vi "Configure9206.vi"(7 "Channel Number":i32, 8 "error in (no error)":errorcluster, 10 "Properties":T1[](array[typedef]), 11 "IO Ref in":refnum<k21>) -> (0 "error out":errorcluster, 3 "IO Ref out":refnum<k21>)   [LabVIEW 2017, in "ScanEngine.lvlib"]
uses:
  <vilib>/addons/InsightCM/Devices/Shared/Common/ScanEngine/ScanEngine.lvlib
  <vilib>/addons/InsightCM/MessageBus/Base/controls/KeyValuePair.ctl
  <resource>/objmgr/cRIO.rc
  <vilib>/addons/InsightCM/Utilities/PropertyHelpers/PropertyHelpers.lvlib
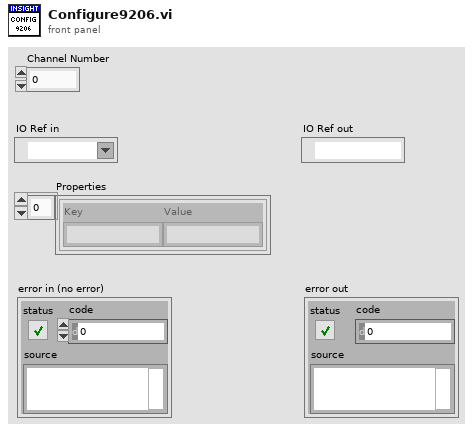
[diagram p1: front panel]
types:
  T1 = typedef "KeyValuePair.ctl" = cluster{"Key":string, "Value":string}
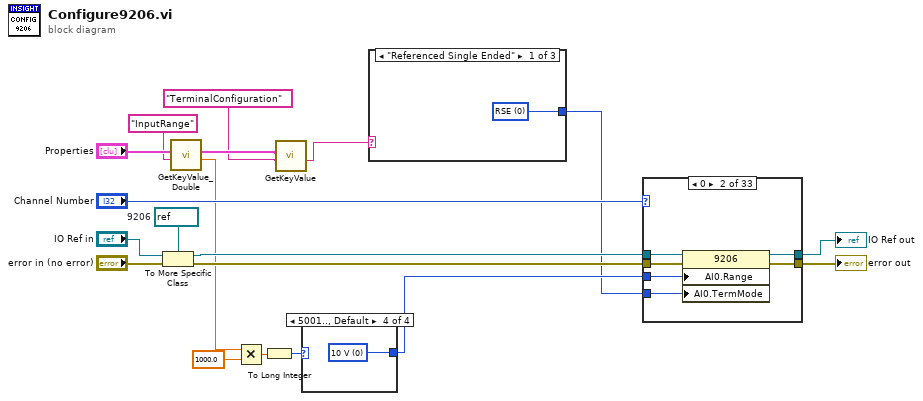
[diagram p0: block diagram]
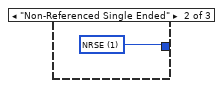
[diagram p2: hidden frame]
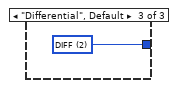
[diagram p3: hidden frame]
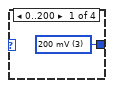
[diagram p4: hidden frame]
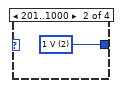
[diagram p5: hidden frame]
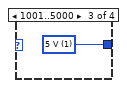
[diagram p6: hidden frame]
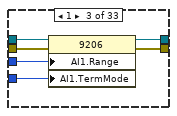
[diagram p8: hidden frame]
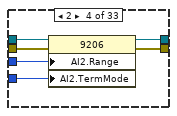
[diagram p9: hidden frame]
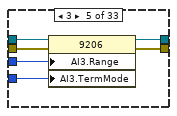
[diagram p10: hidden frame]
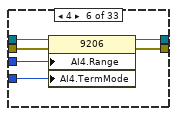
[diagram p11: hidden frame]
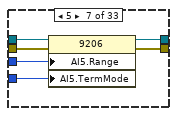
[diagram p12: hidden frame]
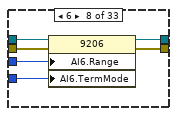
[diagram p13: hidden frame]
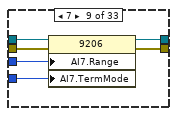
[diagram p14: hidden frame]
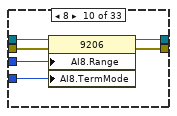
[diagram p15: hidden frame]
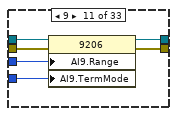
[diagram p16: hidden frame]
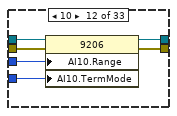
[diagram p17: hidden frame]
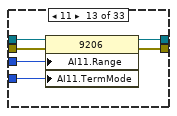
[diagram p18: hidden frame]
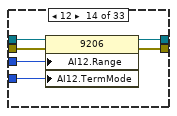
[diagram p19: hidden frame]
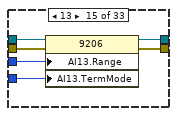
[diagram p20: hidden frame]
diagram:
  w12 = refnum<k21> refnum  # 9206
  n1 = To More Specific Class(target class=w12, reference="IO Ref in", error in="error in (no error)") -> (specific class reference=w11:refnum<k21>, error out=w15:errorcluster)
  n2 = call <vilib>:"GetKeyValue_Double.vi"("key"="InputRange" ("name"), "key value pairs"="Properties") -> ("value"=w5:dbl, "key value pairs out"=w4:T1[])  [unwired: 7 in, 1 out]
  n3 = Multiply(x=w5, y=1000.0) -> (x*y=w17:dbl)
  n4 = To Long Integer(number=w17) -> (32bit integer=w16:i32)
  n5 = call <vilib>:"GetKeyValue.vi"("key"="TerminalConfiguration" ("name"), "key value pairs"=w4) -> ("value"=w2:string)  [unwired: 7 in, 2 out]
  n6 = case shown="5001.., Default" w16 {
    tunnel: [w20 w21 w22 w23] -> w19
    frame 0..200 {
      w20 = u32 3 items=["10 V", "5 V", "1 V", "200 mV"] ("9205 Range")
    }
    frame 201..1000 {
      w21 = u32 2 items=["10 V", "5 V", "1 V", "200 mV"] ("9205 Range")
    }
    frame 1001..5000 {
      w22 = u32 1 items=["10 V", "5 V", "1 V", "200 mV"] ("9205 Range")
    }
    frame 5001.., Default {
      w23 = u32 0 items=["10 V", "5 V", "1 V", "200 mV"] ("9205 Range")
    }
  }
  n7 = case shown="\"Referenced Single Ended\"" w2 {
    tunnel: [w24 w25 w26] -> w1
    frame "Referenced Single Ended" {
      w24 = u32 0 items=["RSE", "NRSE", "DIFF"] ("AI0:Terminal mode")
    }
    frame "Non-Referenced Single Ended" {
      w25 = u32 1 items=["RSE", "NRSE", "DIFF"] ("AI0:Terminal mode")
    }
    frame "Differential", Default {
      w26 = u32 2 items=["RSE", "NRSE", "DIFF"] ("AI0:Terminal mode")
    }
  }
  n8 = case shown="0" "Channel Number" {
    tunnel: w15 -> [w28 w34 w40 w46 w52 w58 w64 w70 w76 w82 w88 w94 w100 w106 w112 w118 w124 w130 w136 w142 w148 w154 w160 w166 w172 w178 w184 w190 w196 w202 w208 w214 w220]
    tunnel: [w28 w33 w39 w45 w51 w57 w63 w69 w75 w81 w87 w93 w99 w105 w111 w117 w123 w129 w135 w141 w147 w153 w159 w165 w171 w177 w183 w189 w195 w201 w207 w213 w219] -> w8
    tunnel: w11 -> [w27 w32 w38 w44 w50 w56 w62 w68 w74 w80 w86 w92 w98 w104 w110 w116 w122 w128 w134 w140 w146 w152 w158 w164 w170 w176 w182 w188 w194 w200 w206 w212 w218]
    tunnel: [w27 w31 w37 w43 w49 w55 w61 w67 w73 w79 w85 w91 w97 w103 w109 w115 w121 w127 w133 w139 w145 w151 w157 w163 w169 w175 w181 w187 w193 w199 w205 w211 w217] -> w13
    tunnel: w1 -> [_ w30 w36 w42 w48 w54 w60 w66 w72 w78 w84 w90 w96 w102 w108 w114 w120 w126 w132 w138 w144 w150 w156 w162 w168 w174 w180 w186 w192 w198 w204 w210 w216]
    tunnel: w19 -> [_ w29 w35 w41 w47 w53 w59 w65 w71 w77 w83 w89 w95 w101 w107 w113 w119 w125 w131 w137 w143 w149 w155 w161 w167 w173 w179 w185 w191 w197 w203 w209 w215]
    frame -1, Default {
    }
    frame 0 {
      n9 = property class="9206"(reference=w32, error in=w34, "AI0.Range"=w29, "AI0.TermMode"=w30) -> (reference out=w31:refnum<k21>, error out=w33:errorcluster)
    }
    frame 1 {
      n10 = property class="9206"(reference=w38, error in=w40, "AI1.Range"=w35, "AI1.TermMode"=w36) -> (reference out=w37:refnum<k21>, error out=w39:errorcluster)
    }
    frame 2 {
      n11 = property class="9206"(reference=w44, error in=w46, "AI2.Range"=w41, "AI2.TermMode"=w42) -> (reference out=w43:refnum<k21>, error out=w45:errorcluster)
    }
    frame 3 {
      n12 = property class="9206"(reference=w50, error in=w52, "AI3.Range"=w47, "AI3.TermMode"=w48) -> (reference out=w49:refnum<k21>, error out=w51:errorcluster)
    }
    frame 4 {
      n13 = property class="9206"(reference=w56, error in=w58, "AI4.Range"=w53, "AI4.TermMode"=w54) -> (reference out=w55:refnum<k21>, error out=w57:errorcluster)
    }
    frame 5 {
      n14 = property class="9206"(reference=w62, error in=w64, "AI5.Range"=w59, "AI5.TermMode"=w60) -> (reference out=w61:refnum<k21>, error out=w63:errorcluster)
    }
    frame 6 {
      n15 = property class="9206"(reference=w68, error in=w70, "AI6.Range"=w65, "AI6.TermMode"=w66) -> (reference out=w67:refnum<k21>, error out=w69:errorcluster)
    }
    frame 7 {
      n16 = property class="9206"(reference=w74, error in=w76, "AI7.Range"=w71, "AI7.TermMode"=w72) -> (reference out=w73:refnum<k21>, error out=w75:errorcluster)
    }
    frame 8 {
      n17 = property class="9206"(reference=w80, error in=w82, "AI8.Range"=w77, "AI8.TermMode"=w78) -> (reference out=w79:refnum<k21>, error out=w81:errorcluster)
    }
    frame 9 {
      n18 = property class="9206"(reference=w86, error in=w88, "AI9.Range"=w83, "AI9.TermMode"=w84) -> (reference out=w85:refnum<k21>, error out=w87:errorcluster)
    }
    frame 10 {
      n19 = property class="9206"(reference=w92, error in=w94, "AI10.Range"=w89, "AI10.TermMode"=w90) -> (reference out=w91:refnum<k21>, error out=w93:errorcluster)
    }
    frame 11 {
      n20 = property class="9206"(reference=w98, error in=w100, "AI11.Range"=w95, "AI11.TermMode"=w96) -> (reference out=w97:refnum<k21>, error out=w99:errorcluster)
    }
    frame 12 {
      n21 = property class="9206"(reference=w104, error in=w106, "AI12.Range"=w101, "AI12.TermMode"=w102) -> (reference out=w103:refnum<k21>, error out=w105:errorcluster)
    }
    frame 13 {
      n22 = property class="9206"(reference=w110, error in=w112, "AI13.Range"=w107, "AI13.TermMode"=w108) -> (reference out=w109:refnum<k21>, error out=w111:errorcluster)
    }
    frame 14 {
      n23 = property class="9206"(reference=w116, error in=w118, "AI14.Range"=w113, "AI14.TermMode"=w114) -> (reference out=w115:refnum<k21>, error out=w117:errorcluster)
    }
    frame 15 {
      n24 = property class="9206"(reference=w122, error in=w124, "AI15.Range"=w119, "AI15.TermMode"=w120) -> (reference out=w121:refnum<k21>, error out=w123:errorcluster)
    }
    frame 16 {
      n25 = property class="9206"(reference=w128, error in=w130, "AI16.Range"=w125, "AI16.TermMode"=w126) -> (reference out=w127:refnum<k21>, error out=w129:errorcluster)
    }
    frame 17 {
      n26 = property class="9206"(reference=w134, error in=w136, "AI17.Range"=w131, "AI17.TermMode"=w132) -> (reference out=w133:refnum<k21>, error out=w135:errorcluster)
    }
    frame 18 {
      n27 = property class="9206"(reference=w140, error in=w142, "AI18.Range"=w137, "AI18.TermMode"=w138) -> (reference out=w139:refnum<k21>, error out=w141:errorcluster)
    }
    frame 19 {
      n28 = property class="9206"(reference=w146, error in=w148, "AI19.Range"=w143, "AI19.TermMode"=w144) -> (reference out=w145:refnum<k21>, error out=w147:errorcluster)
    }
    frame 20 {
      n29 = property class="9206"(reference=w152, error in=w154, "AI20.Range"=w149, "AI20.TermMode"=w150) -> (reference out=w151:refnum<k21>, error out=w153:errorcluster)
    }
    frame 21 {
      n30 = property class="9206"(reference=w158, error in=w160, "AI21.Range"=w155, "AI21.TermMode"=w156) -> (reference out=w157:refnum<k21>, error out=w159:errorcluster)
    }
    frame 22 {
      n31 = property class="9206"(reference=w164, error in=w166, "AI22.Range"=w161, "AI22.TermMode"=w162) -> (reference out=w163:refnum<k21>, error out=w165:errorcluster)
    }
    frame 23 {
      n32 = property class="9206"(reference=w170, error in=w172, "AI23.Range"=w167, "AI23.TermMode"=w168) -> (reference out=w169:refnum<k21>, error out=w171:errorcluster)
    }
    frame 24 {
      n33 = property class="9206"(reference=w176, error in=w178, "AI24.Range"=w173, "AI24.TermMode"=w174) -> (reference out=w175:refnum<k21>, error out=w177:errorcluster)
    }
    frame 25 {
      n34 = property class="9206"(reference=w182, error in=w184, "AI25.Range"=w179, "AI25.TermMode"=w180) -> (reference out=w181:refnum<k21>, error out=w183:errorcluster)
    }
    frame 26 {
      n35 = property class="9206"(reference=w188, error in=w190, "AI26.Range"=w185, "AI26.TermMode"=w186) -> (reference out=w187:refnum<k21>, error out=w189:errorcluster)
    }
    frame 27 {
      n36 = property class="9206"(reference=w194, error in=w196, "AI27.Range"=w191, "AI27.TermMode"=w192) -> (reference out=w193:refnum<k21>, error out=w195:errorcluster)
    }
    frame 28 {
      n37 = property class="9206"(reference=w200, error in=w202, "AI28.Range"=w197, "AI28.TermMode"=w198) -> (reference out=w199:refnum<k21>, error out=w201:errorcluster)
    }
    frame 29 {
      n38 = property class="9206"(reference=w206, error in=w208, "AI29.Range"=w203, "AI29.TermMode"=w204) -> (reference out=w205:refnum<k21>, error out=w207:errorcluster)
    }
    frame 30 {
      n39 = property class="9206"(reference=w212, error in=w214, "AI30.Range"=w209, "AI30.TermMode"=w210) -> (reference out=w211:refnum<k21>, error out=w213:errorcluster)
    }
    frame 31 {
      n40 = property class="9206"(reference=w218, error in=w220, "AI31.Range"=w215, "AI31.TermMode"=w216) -> (reference out=w217:refnum<k21>, error out=w219:errorcluster)
    }
  }
  "IO Ref out" <- w13
  "error out" <- w8
